vi "OAT Output Triggered Even Angle Signal.vi"   [LabVIEW 2017, in "SoundVib_OAUtility.lvlib"]
doc: "Generates triggered even-angle signals for vector averaging in order power spectrum calculations. Use this VI to remove uncorrelated phenomenon for vector averaging. Each instance of this VI maintains its own state; use the N Waveforms instance of this VI to process an array of channels. Wire data to the <B>even-angle signal</B> input to determine the polymorphic instance to use or manually select the instance."
uses:
  <vilib>/addons/Sound and Vibration/Order Analysis/Utility/SoundVib_OAUtility.lvlib
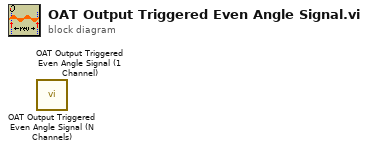
[diagram p0: block diagram]
diagram:
  n1 = call <vilib>:"OAT Output Triggered Even Angle Signal (N Channels).vi"() -> ()  [unwired: 13 in, 3 out]
  n2 = call <vilib>:"OAT Output Triggered Even Angle Signal (1 Channel).vi"() -> ()  [unwired: 13 in, 3 out]
